vi "Unpack DPad.vi"(11 "Axes":T1) -> (0 "Right":bool, 1 "Left":bool, 2 "Down":bool, 3 "Up":bool)   [LabVIEW 2013]
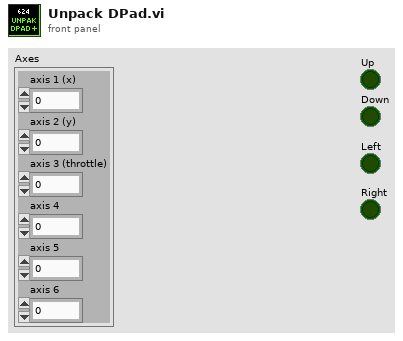
[diagram p1: front panel]
types:
  T1 = cluster{"axis 1 (x)":dbl, "axis 2 (y)":dbl, "axis 3 (throttle)":dbl, "axis 4":dbl, "axis 5":dbl, "axis 6":dbl}
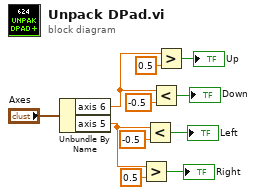
[diagram p0: block diagram]
diagram:
  n1 = Unbundle By Name("Axes") -> ("axis 6"=w6:dbl, "axis 5"=w9:dbl)
  n2 = Greater?(x=w9, y=0.5) -> (0:→"Right":bool)
  n3 = Less?(x=w9, y=-0.5) -> (x < y?=→"Left":bool)
  n4 = Less?(x=w6, y=-0.5) -> (x < y?=→"Down":bool)
  n5 = Greater?(x=w6, y=0.5) -> (0:→"Up":bool)
